vi "FM Modulation Demo (Single tone) - First.vi"() -> ()   [LabVIEW 2013]
uses:
  <vilib>/express/express analysis/Spectral/Block/exnSpectralBlock spectral measurements power poly.vi
  <vilib>/express/express analysis/Spectral/Block/exnSpectralBlock spectral measurements power DDT.vi
  <vilib>/express/express analysis/Spectral/XNode/ExpressSpectralMeasurementsBlockNode.xnode
panel:
  in  "WAV Sample Rate":dbl=44100.0 caption="dt"
  in  "Mod. Freq.":dbl=2000.0 caption="Frequency"
  in  "LPF Cut-Off":dbl=10000.0 caption="Lower Cut-Off"
  in  "AWGN (dB)":dbl(slide)=0.6 caption="Standard deviation" scale=-20.0..30.0
  out "Comparision":dynamicdata(graph)
  out "Baseband":dynamicdata(graph)
  out "FM FFT":dynamicdata(graph)
  out "FM Wave":dynamicdata(graph)
  in  "DC Offset":dbl=1.0
  in  "Carrier Amp.":dbl=1.0 caption="Amplitude"
  in  "stop":bool
  in  "Frequency Deviation":dbl(slide)=1.0 scale=0.0..5.0
  in  "Carrier Freq.":dbl=100000.0 caption="Frequency"
  out "After Rectifier":cluster{"f0":dbl, "df":dbl, "magnitude":dbl[]}(graph)
  # "FM Modulation"
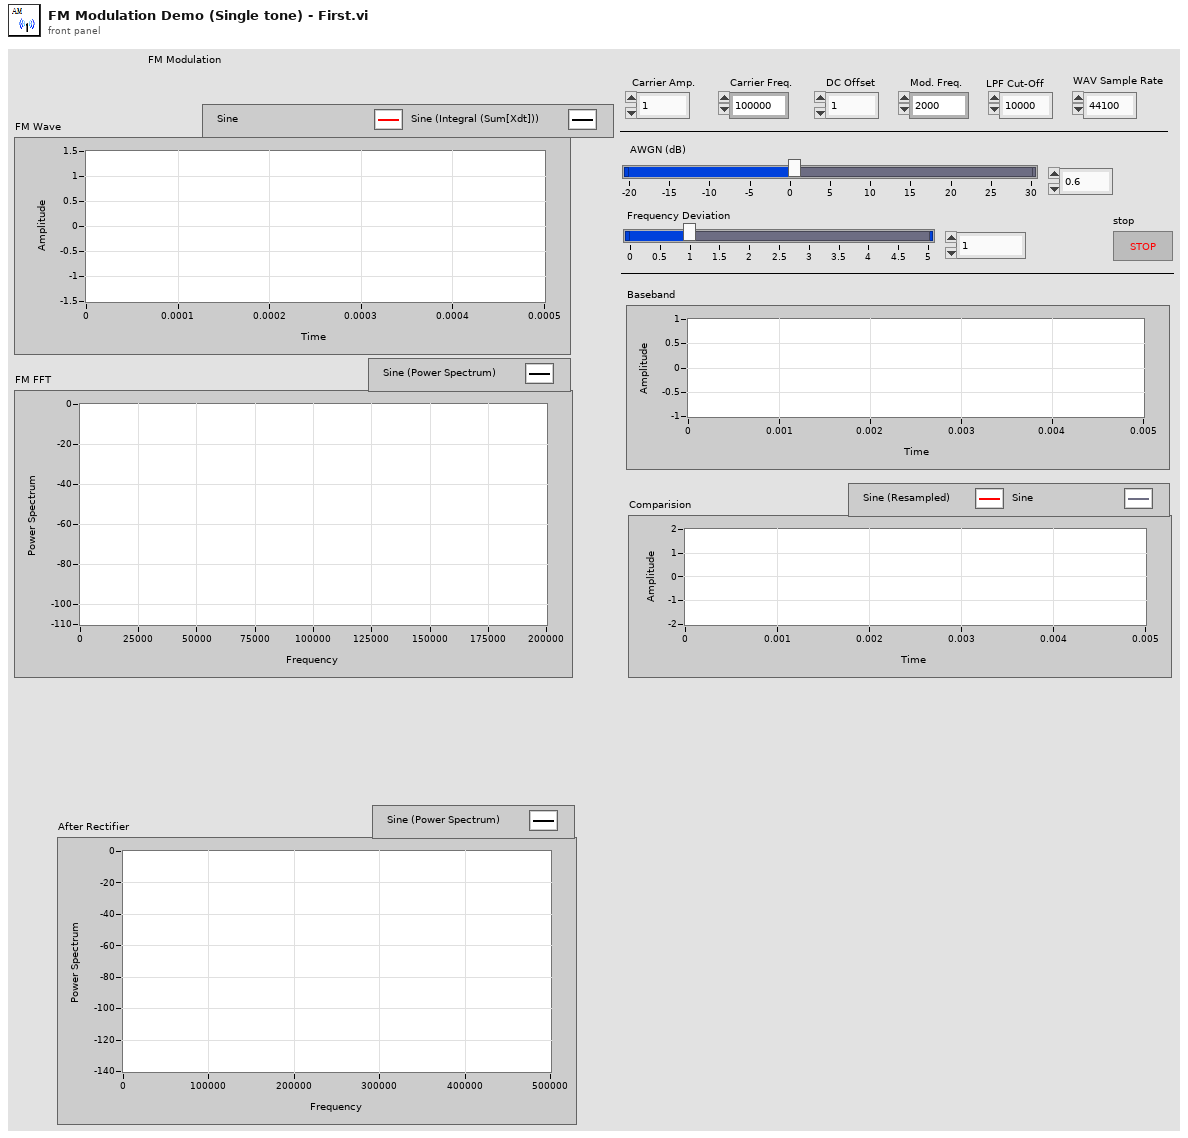
[diagram p1: front panel]
types:
  T1 = cluster{"averaging mode":u16, "weighting mode":u16, "number of averages":u32}
  T2 = cluster{"dB On (F)":bool, "unwrap phase (F)":bool, "convert to degree (F)":bool}
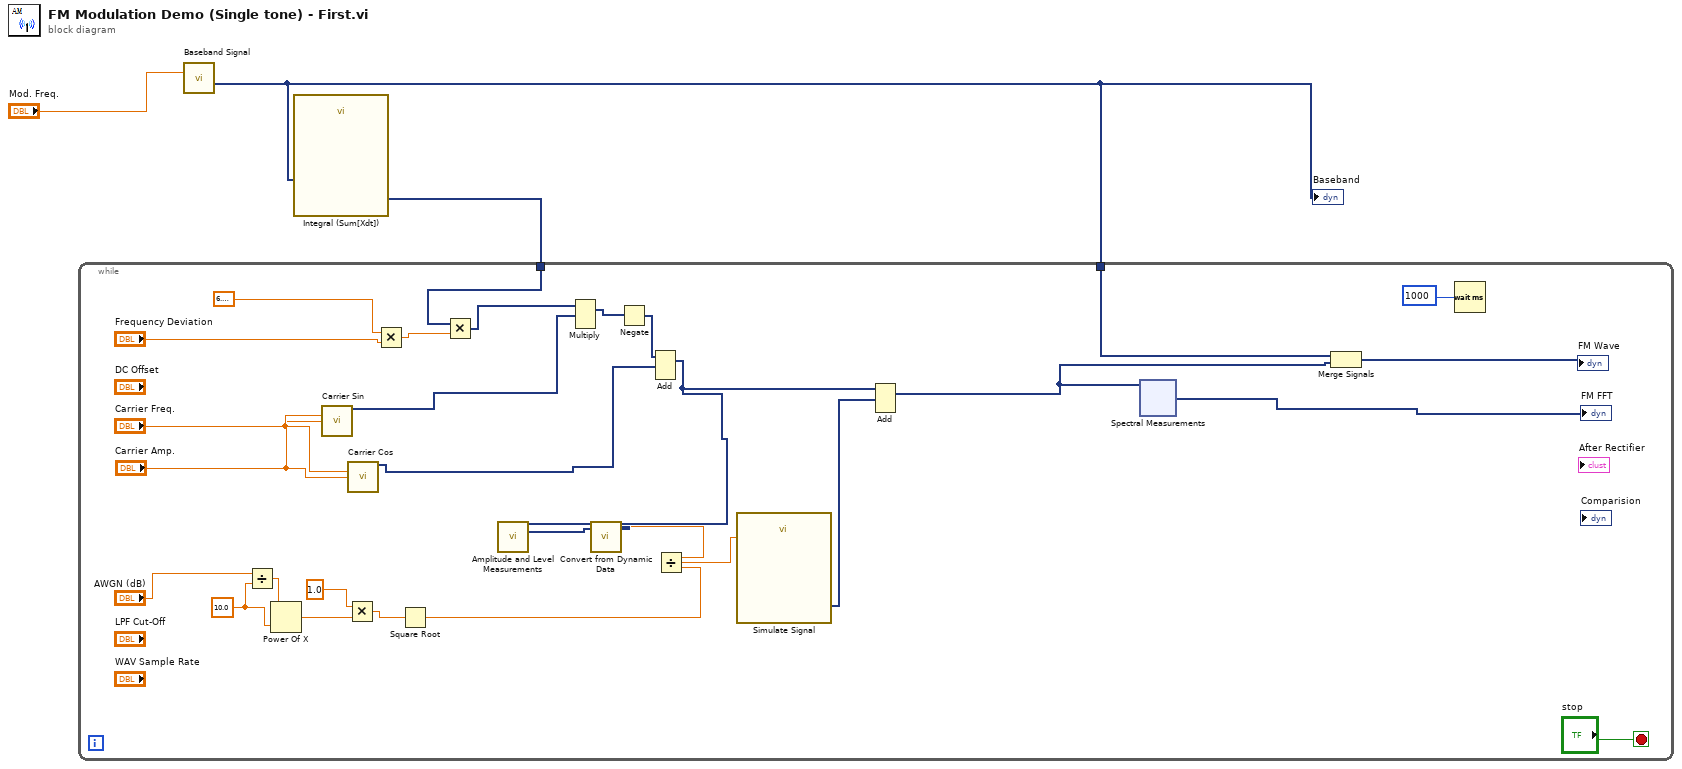
[diagram p0: block diagram]
diagram:
  n1 = call "Baseband Signal"("Frequency"="Mod. Freq.") -> ("Sine"=w2:dynamicdata)  [unwired: 13 in, 1 out]
  "Baseband" <- w2
  n2 = call "Integral (Sum[Xdt])"("Signals"=w2) -> ("Result"=w1:dynamicdata)  [unwired: 5 in, 1 out]
  n3 = while {
    tunnel: w2 -> [w9]
    tunnel: w1 -> [w13]
    stop <- "stop" stop-if-true
    w18 = 10.0
    n4 = Divide(x="AWGN (dB)", y=w18) -> (x/y=w19:dbl)
    n5 = Power Of X(1:w18, 2:w19) -> (0:w17:dbl)
    n6 = call "Carrier Sin"("Frequency"="Carrier Freq.", "Amplitude"="Carrier Amp.") -> ("Sine"=w8:dynamicdata)  [unwired: 12 in, 1 out]
    n7 = Multiply(x=1.0, y=w17) -> (x*y=w26:dbl)
    n8 = call "Carrier Cos"("Frequency"="Carrier Freq.", "Amplitude"="Carrier Amp.") -> ("Sine"=w6:dynamicdata)  [unwired: 12 in, 1 out]
    n9 = Multiply(x=6.283185307179586, y="Frequency Deviation") -> (x*y=w14:dbl)
    n10 = Square Root(x=w26) -> (sqrt(x)=w24:dbl)
    n11 = Multiply(x=w13, y=w14) -> (x*y=w7:dynamicdata)
    n12 = Multiply(1:w8, 2:w7) -> (0:w5:dynamicdata)  [unwired: 1 in, 1 out]
    n13 = Negate(x=w5) -> (-x=w4:dynamicdata)
    n14 = Add(1:w6, 2:w4) -> (0:w10:dynamicdata)  [unwired: 1 in, 1 out]
    n15 = call "Amplitude and Level Measurements"("Signals"=w10) -> ("RMS"=w29:dynamicdata)  [unwired: 13 in, 1 out]
    n16 = call "Convert from Dynamic Data"("Dynamic Data Type"=w29) -> ("Scalar"=w25:dbl)  [unwired: 3 in]
    n17 = Divide(x=w25, y=w24) -> (x/y=w16:dbl)
    n18 = call "Simulate Signal"("Standard deviation"=w16) -> ("DC with Gaussian Noise"=w23:dynamicdata)  [unwired: 13 in, 1 out]
    n19 = Add(1:w23, 2:w10) -> (0:w22:dynamicdata)  [unwired: 1 in, 1 out]
    n20 = xnode "Spectral Measurements"("Signals"=w22) -> ("Power Spectrum"=→"FM FFT":dynamicdata)  [unwired: 1 in, 1 out]
    n21 = Merge Signals(w9, w22) -> (→"FM Wave":dynamicdata)
    n22 = Wait (ms)(milliseconds to wait=1000) -> ()  [unwired: 1 out]
  }
